vi "Set Voltage.vi"(8 "error in":errorcluster, 10 "Voltage":sgl, 11 "SR 3XX HVPS in":refnum<class "SR 3XX HVPS.lvclass">) -> (0 "error out":errorcluster, 3 "SR 3XX HVPS out":refnum<class "SR 3XX HVPS.lvclass">)   [LabVIEW 2014, in "SR 3XX HVPS.lvclass"]
doc: "The VSET command sets the value of the voltage set to x if front panel control is enabled. If rear panel control is enabled, an error is returned. The value x is a number in the units of Volts and the sign of the number MUST match the PS300’s polarity setting.As with front panel control, the VSET value must be less than or equal to to VLIM value or an execution error will be returned."
uses:
  SR 3XX HVPS.lvclass
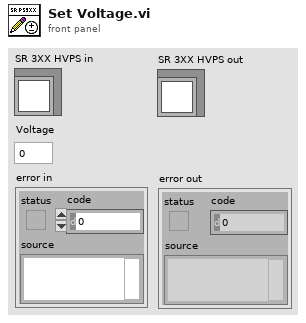
[diagram p1: front panel]
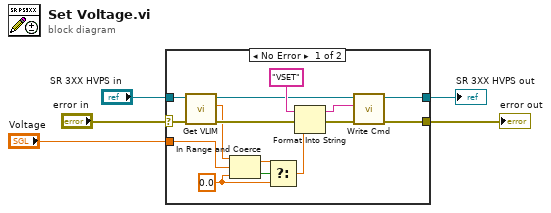
[diagram p0: block diagram]
diagram:
  n1 = case shown="No Error" "error in" {
    selector: "error in" -> [w16 w22]
    tunnel: [w6 w22] -> w4
    tunnel: [w7 w21] -> w2
    tunnel: "SR 3XX HVPS in" -> [w17 w21]
    tunnel: "Voltage" -> [w10 _]
    frame No Error {
      w11 = sgl 0.0 ("lower limit")
      n2 = call "Get VLIM.vi"("error in"=w16, "SR 3XX HVPS in"=w17) -> ("error out"=w14:errorcluster, "VLIM"=w13:sgl, "SR 3XX HVPS out"=w15:refnum<class "SR 3XX HVPS.lvclass">)  [unwired: 7 in]
      n3 = In Range and Coerce(upper limit=w13, x=w10, lower limit=w11) -> (coerced(x)=w8:sgl, In Range?=w12:bool)
      n4 = Select(t=w8, s=w12, f=w11) -> (s? t:f=w9:sgl)
      n5 = Format Into String(initial string="VSET", error in=w14, w9) -> (resulting string=w19:string, error out=w18:errorcluster)  [unwired: 1 in]
      n6 = call "Write Cmd.vi"("error in"=w18, "Cmd"=w19, "SR 3XX HVPS in"=w15) -> ("error out"=w6:errorcluster, "SR 3XX HVPS out"=w7:refnum<class "SR 3XX HVPS.lvclass">)  [unwired: 7 in]
    }
    frame Error {
    }
  }
  "error out" <- w4
  "SR 3XX HVPS out" <- w2
